vi "Proyecto.vi"() -> ()   [LabVIEW 2020]
uses:
  <vilib>/Instr/_visa.llb/VISA Configure Serial Port (Instr).vi
panel:
  out "ACTUADOR":bool
  out "VÁLVULA 75% ABIERTA":bool
  out "CODO 4":bool
  out "CODO 3":bool
  in  "?":enum32{"Control y visualización"}(tab)
  out "Waveform Chart":dbl(graph)
  in  "Nivel de altura deseada":dbl(slide) scale=0.0..22.5
  in  "Puerto de conexión con Arduino":refnum<visa-resource-name>
  in  "STOP":bool
  out "Altura":dbl
  out "TANQUE 2":i8(slide) scale=0.0..36.0
  in  "TUBERIA 7":u8(slide) scale=0.0..20.0
  out "VÁLVULA 100% ABIERTA":bool
  in  "TUBERIA 6":u8(slide) scale=0.0..20.0
  out "TANQUE 1":i8(slide) scale=0.0..36.0
  in  "TUBERIA 5":u8(slide) scale=0.0..20.0
  in  "TUBERIA 4":u8(slide) scale=0.0..20.0
  out "PWM motor":dbl
  out "Control":dbl
  # "Unidad Profesional Interdisciplinaria de Ingeniería Campus Zacatecas\nInstituto Politécnico Nacional"
  # "Unidad Profesional Interdisciplinaria de Ingeniería Campus Zacatecas\nInstituto Politécnico Nacional"
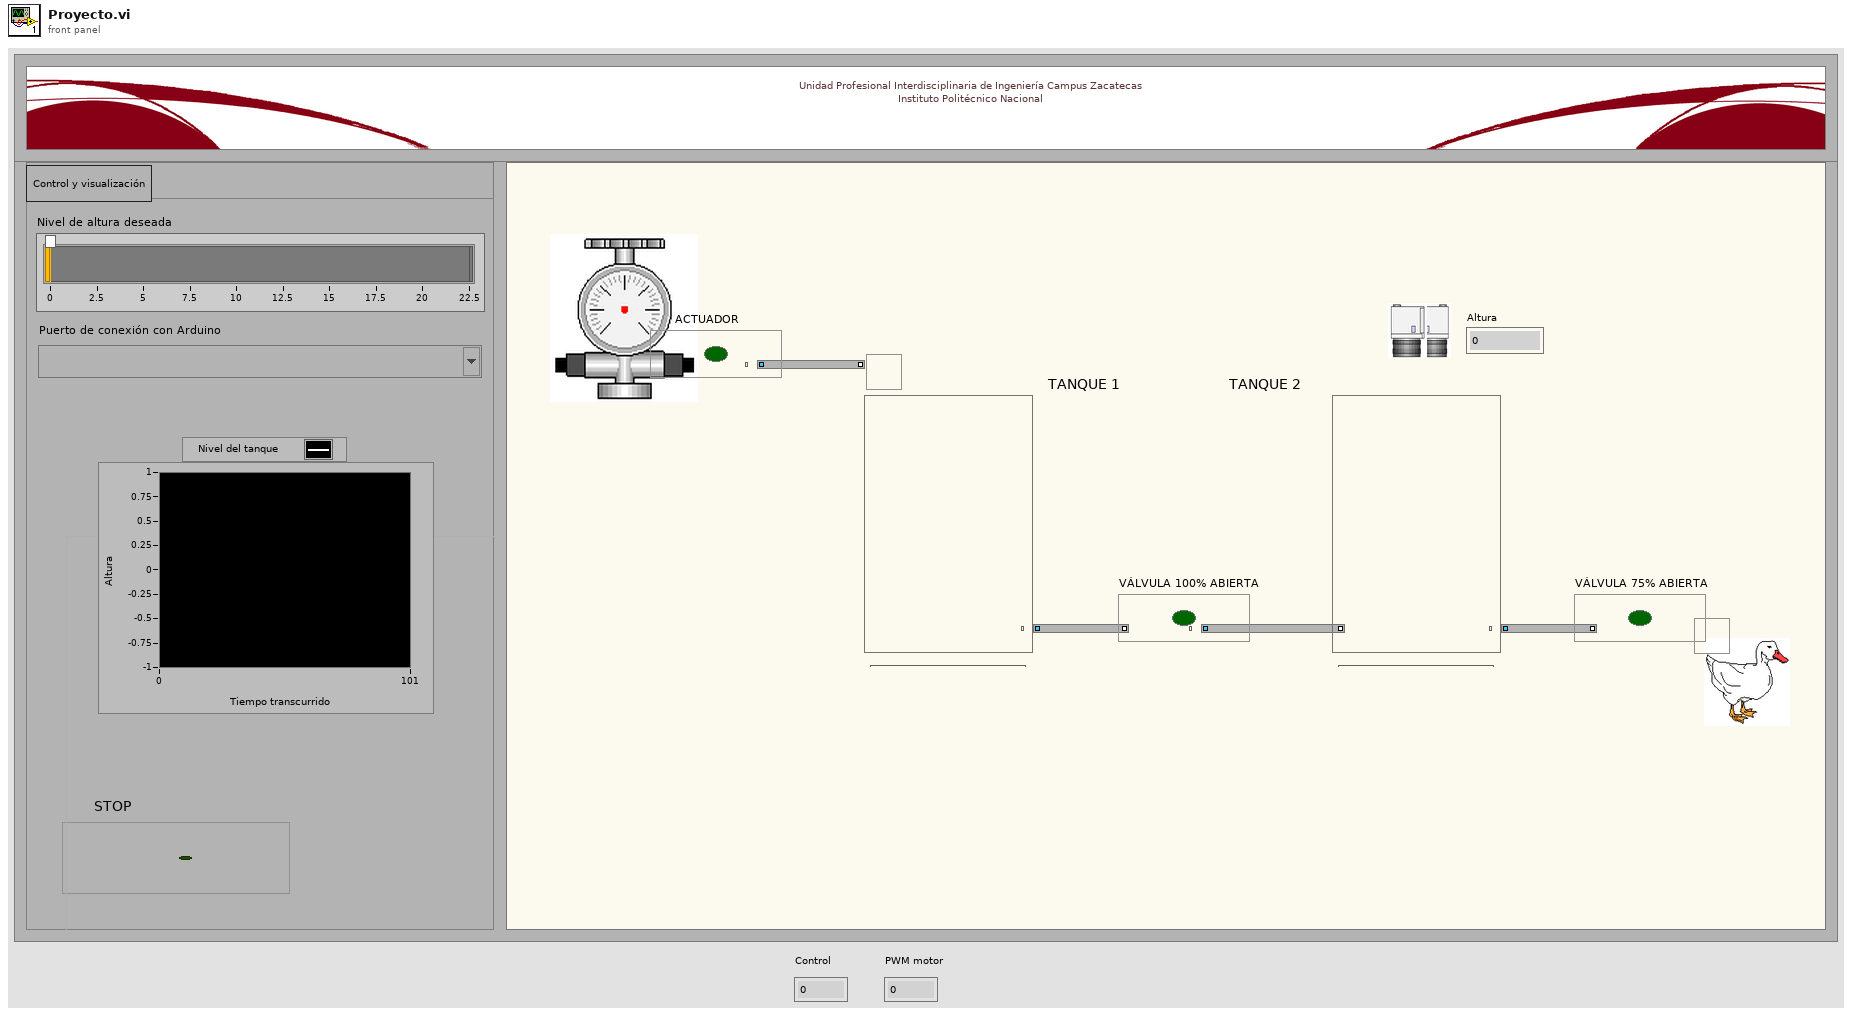
[diagram p1: front panel]
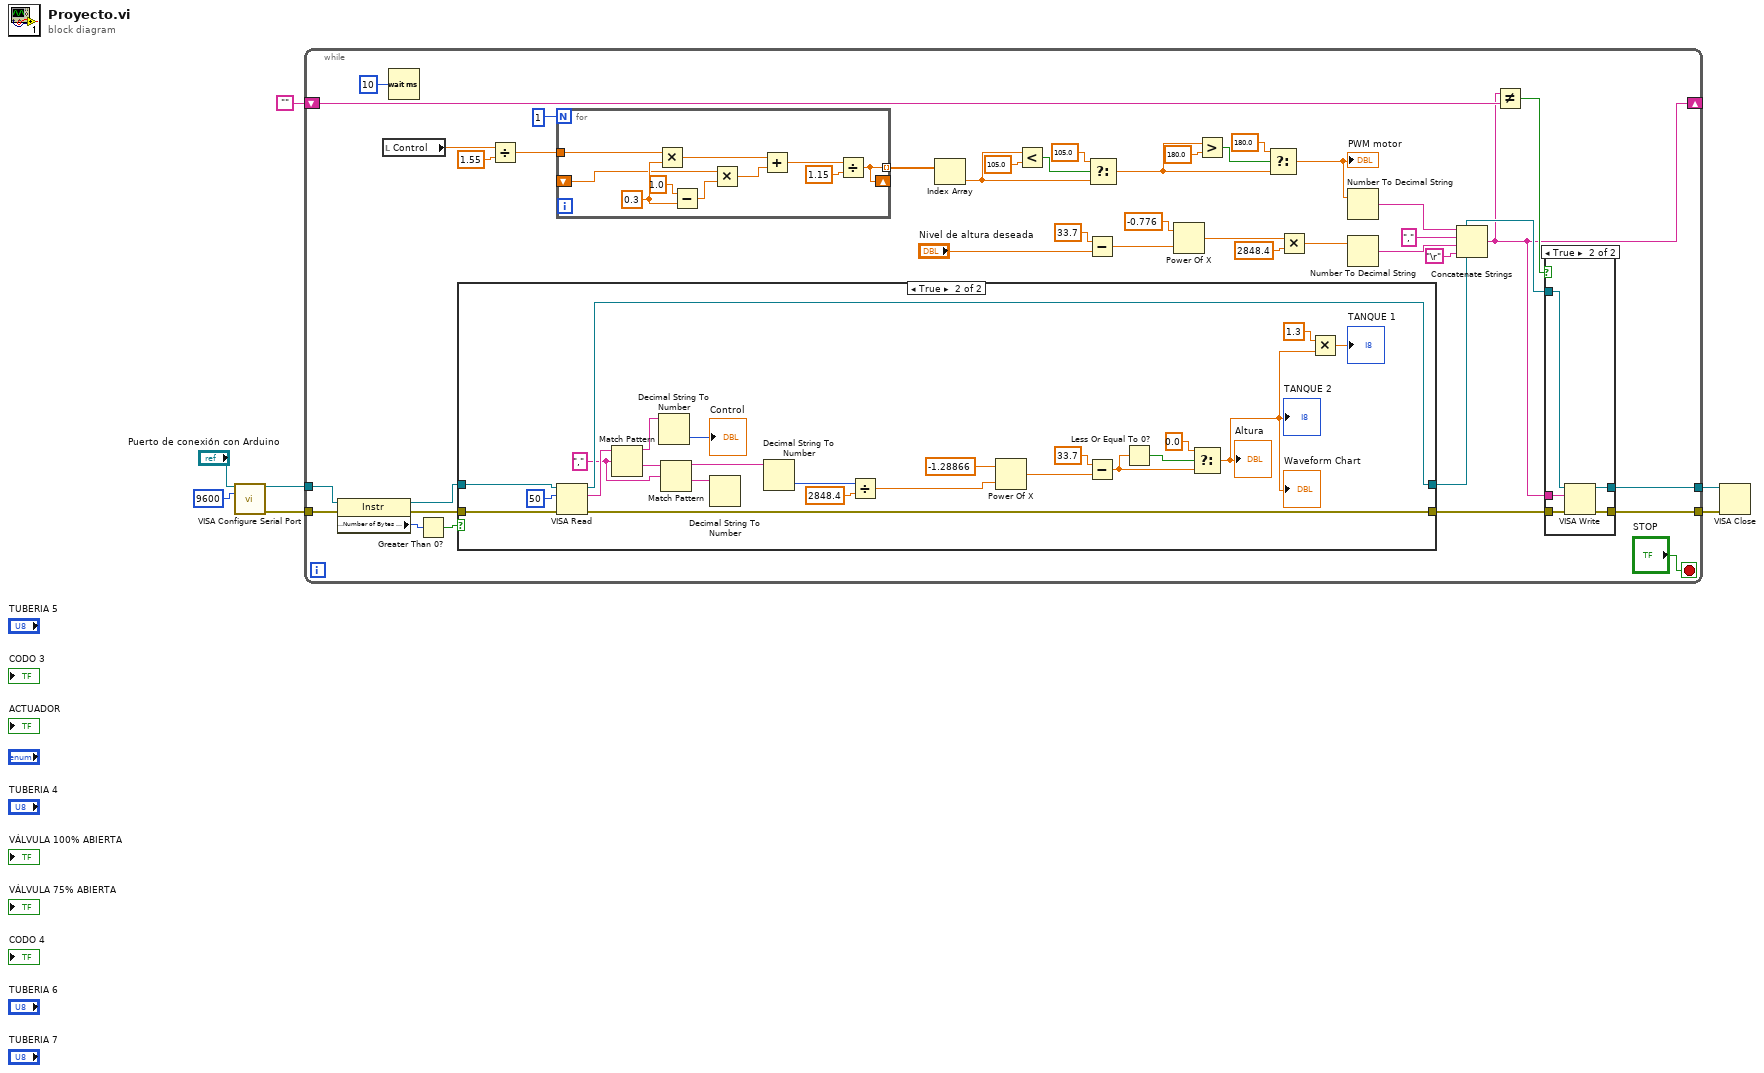
[diagram p0: block diagram]
diagram:
  n1 = call-poly "VISA Configure Serial Port"("VISA resource name"="Puerto de conexión con Arduino", "baud rate (9600)"=u32 9600) -> ("VISA resource name out"=w7:refnum<visa-resource-name>, "error out"=w4:errorcluster)  [unwired: 12 in]
  n2 = while {
    tunnel: w7 -> [w46]
    tunnel: w4 -> [w45]
    tunnel: [w39] -> w3
    tunnel: [w38] -> w2
    shift-right: [w34] -> _
    shift-left: "" -> [w36]
    stop <- "STOP" stop-if-true
    n3 = property class="Instr"(reference=w46, error in=w45) -> (reference out=w47:refnum<visa-resource-name>, error out=w44:errorcluster, "Serial Settings:Number of Bytes at Serial Port"=w42:u32)
    n4 = local read "Control"() -> (w33:dbl)
    n5 = Wait (ms)(milliseconds to wait=u32 10) -> ()  [unwired: 1 out]
    n6 = Greater Than 0?(x=w42) -> (x > 0?=w43:bool)
    n7 = case shown="True" w43 {
      tunnel: w47 -> [w66 w90]
      tunnel: [w66 w89] -> w41
      tunnel: w44 -> [w65 w88]
      tunnel: [w65 w87] -> w40
      frame False {
      }
      frame True {
        w81 = "," ("regular expression")
        n8 = VISA Read(VISA resource name=w90, byte count=50, error in (no error)=w88) -> (VISA resource name out=w89:refnum<visa-resource-name>, read buffer=w84:string, error out=w87:errorcluster)  [unwired: 1 out]
        n9 = Match Pattern(string=w84, regular expression=w81) -> (before substring=w83:string, after substring=w82:string)  [unwired: 1 in, 2 out]
        n10 = Decimal String To Number(string=w83) -> (number=→"Control":i32)  [unwired: 2 in, 1 out]
        n11 = Match Pattern(string=w82, regular expression=w81) -> (before substring=w80:string, after substring=w79:string)  [unwired: 1 in, 2 out]
        n12 = Decimal String To Number(string=w79) -> ()  [unwired: 2 in, 2 out]
        n13 = Decimal String To Number(string=w80) -> (number=w75:i32)  [unwired: 2 in, 1 out]
        n14 = Divide(x=w75, y=2848.4) -> (x/y=w74:dbl)
        n15 = Power Of X(1:w74, 2:-1.28866 ("y")) -> (0:w71:dbl)
        n16 = Subtract(x=33.7, y=w71) -> (x-y=w67:dbl)
        n17 = Less Or Equal To 0?(x=w67) -> (x <= 0?=w70:bool)
        n18 = Select(t=0.0, s=w70, f=w67) -> (s? t:f=w68:dbl)
        "TANQUE 2" <- w68
        "Altura" <- w68
        "Waveform Chart" <- w68
        n19 = Multiply(x=1.3, y=w68) -> (x*y=→"TANQUE 1":dbl)
      }
    }
    n20 = Divide(x=w33, y=1.55) -> (x/y=w11:dbl)
    n21 = for {
      N: 1 -> [_]
      tunnel: w11 -> [w52]
      shift-right: [w48] -> _
      shift-left: _ -> [w51]
      tunnel: [w48] -> w10 mode=indexing
      w54 = 0.3 ("y")
      n22 = Multiply(x=w52, y=w54) -> (x*y=w57:dbl)
      n23 = Subtract(x=1.0, y=w54) -> (x-y=w56:dbl)
      n24 = Multiply(x=w51, y=w56) -> (x*y=w53:dbl)
      n25 = Add(x=w57, y=w53) -> (x+y=w50:dbl)
      n26 = Divide(x=w50, y=1.15) -> (x/y=w48:dbl)
    }
    n27 = Index Array(array=w10) -> (element=w18:dbl)  [unwired: 1 in]
    n28 = Less?(x=w18, y=105.0) -> (x < y?=w21:bool)
    n29 = Subtract(x=33.7, y="Nivel de altura deseada") -> (x-y=w26:dbl)
    n30 = Select(t=105.0, s=w21, f=w18) -> (s? t:f=w14:dbl)
    n31 = Power Of X(1:w26, 2:-0.776 ("y")) -> (0:w24:dbl)
    n32 = Greater?(x=w14, y=180.0) -> (0:w16:bool)
    n33 = Select(t=180.0, s=w16, f=w14) -> (s? t:f=w13:dbl)
    "PWM motor" <- w13
    n34 = Multiply(x=w24, y=2848.4) -> (x*y=w22:dbl)
    n35 = Number To Decimal String(number=w13) -> (decimal integer string=w37:string)  [unwired: 1 in]
    n36 = Number To Decimal String(number=w22) -> (decimal integer string=w31:string)  [unwired: 1 in]
    n37 = Concatenate Strings(w37, ",", w31, "\r") -> (w34:string)
    n38 = Not Equal?(x=w34, y=w36) -> (x != y?=w35:bool)
    n39 = case shown="True" w35 {
      tunnel: w41 -> [w59 w64]
      tunnel: w40 -> [w58 w63]
      tunnel: [w59 w62] -> w39
      tunnel: [w58 w61] -> w38
      tunnel: w34 -> [_ w60]
      frame False {
      }
      frame True {
        n40 = VISA Write(VISA resource name=w64, write buffer=w60, error in (no error)=w63) -> (VISA resource name out=w62:refnum<visa-resource-name>, error out=w61:errorcluster)  [unwired: 1 out]
      }
    }
  }
  n41 = VISA Close(VISA resource name=w3, error in (no error)=w2) -> ()  [unwired: 1 out]
